vi "ParamControl.vi"(3 "Time Duration(ms)":i32, 4 "Packet":T1, 6 "Channel Array In":T2(array[cluster])) -> (1 "Ratio":dbl[](array[numeric]), 2 "Channel Array Out":T2(array[cluster]))   [LabVIEW 2014]
panel:
  out "Tmp Ratio":dbl[](array[numeric])
  out "Tmp Delay":dbl[](array[numeric])
  out "delta":dbl
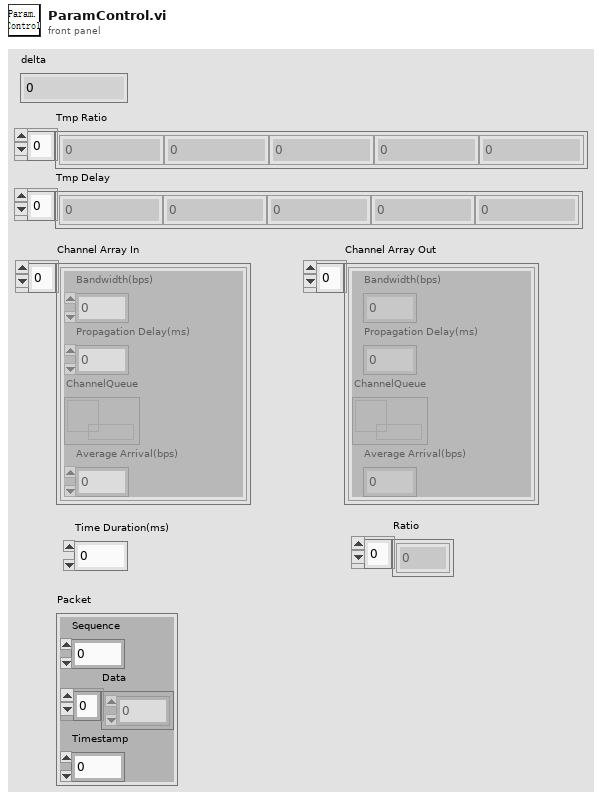
[diagram p1: front panel]
types:
  T1 = cluster{"Sequence":i32, "Data":u8[], "Timestamp":i32}
  T2 = cluster{"Bandwidth(bps)":i32, "Propagation Delay(ms)":i32, "ChannelQueue":refnum<queue>, "Average Arrival(bps)":dbl}[]
  T3 = cluster{"Bandwidth(bps)":i32, "Propagation Delay(ms)":i32, "ChannelQueue":refnum<queue>, "Average Arrival(bps)":dbl}
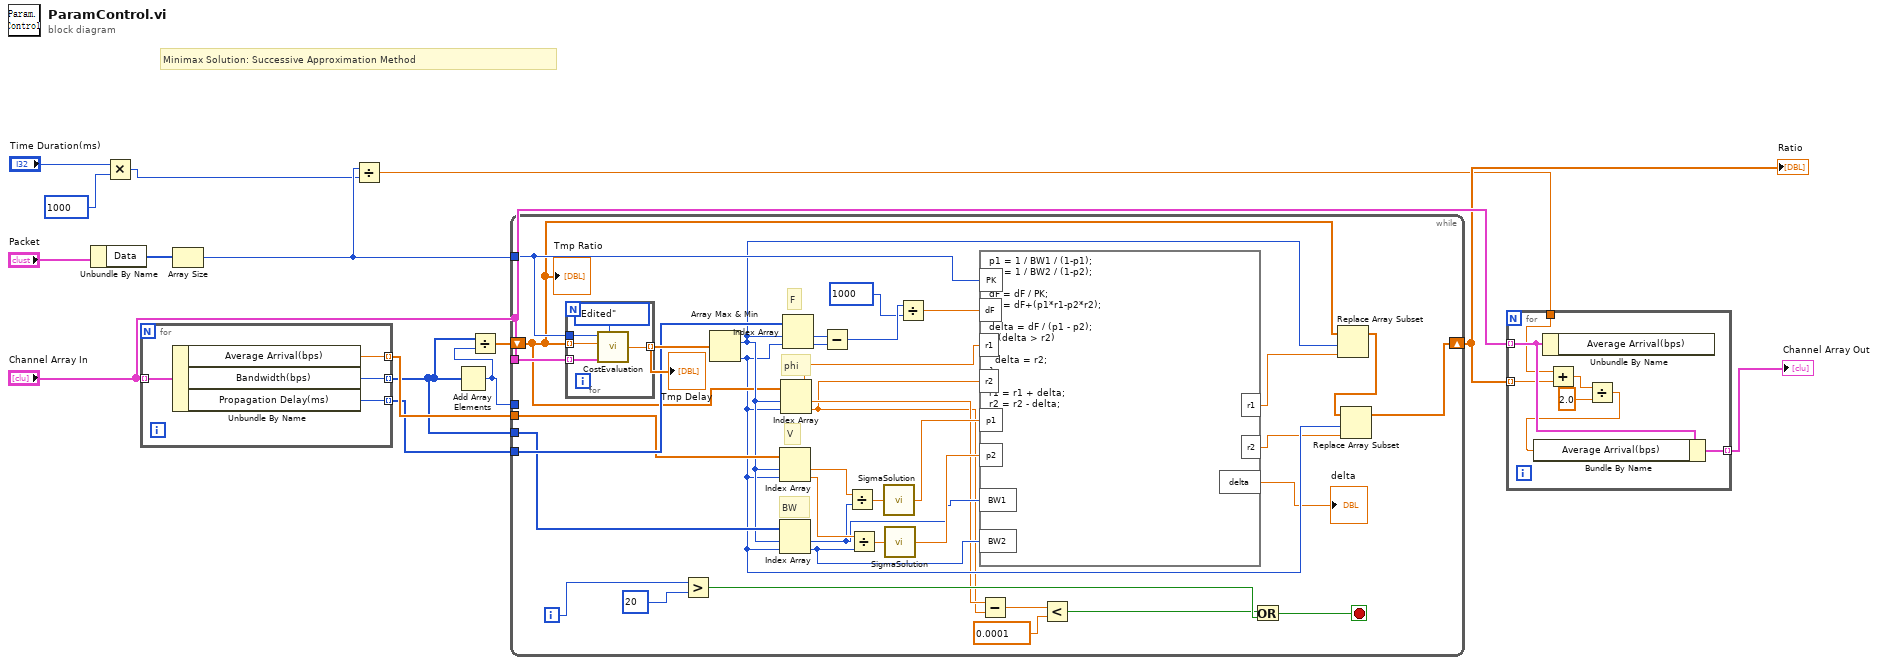
[diagram p0: block diagram]
diagram:
  # "Minimax Solution: Successive Approximation Method"
  n1 = Unbundle By Name("Packet") -> ("Data"=w15:u8[])
  n2 = Multiply(x="Time Duration(ms)", y=1000) -> (x*y=w5:i32)
  n3 = for {
    tunnel: "Channel Array In" -> [w19] mode=indexing
    tunnel: [w18] -> w13 mode=indexing
    tunnel: [w17] -> w12 mode=indexing
    tunnel: [w16] -> w11 mode=indexing
    n4 = Unbundle By Name(w19) -> ("Average Arrival(bps)"=w18:dbl, "Bandwidth(bps)"=w17:i32, "Propagation Delay(ms)"=w16:i32)
  }
  n5 = Array Size(array=w15) -> (size(s)=w6:i32)
  n6 = Divide(x=w6, y=w5) -> (x/y=w2:dbl)
  n7 = Add Array Elements(numeric array=w12) -> (sum=w10:i32)
  n8 = Divide(x=w12, y=w10) -> (x/y=w14:dbl[])
  n9 = while {
    tunnel: w6 -> [w40]
    tunnel: "Channel Array In" -> [w52]
    tunnel: w13 -> [w46]
    tunnel: w12 -> [w45]
    tunnel: w11 -> [w49]
    shift-right: [w28] -> w3
    shift-left: w14 -> [w33]
    tunnel: w10 -> [_]
    i -> [w55]
    stop <- w50 stop-if-true
    # "BW"
    # "V"
    # "phi"
    # "F"
    n10 = for {
      tunnel: w33 -> [w60] mode=indexing
      tunnel: w40 -> [w59]
      tunnel: w52 -> [w58] mode=indexing
      tunnel: [w57] -> w51 mode=indexing
      n11 = call "CostEvaluation.vi"("Packet Size"=w59, "Ratio"=w60, "Channel"=w58, "method"=enum16{"Edited", "original"}."Edited") -> ("delay(s)"=w57:dbl)  [unwired: 1 in]
    }
    "Tmp Delay" <- w51
    n12 = Greater?(x=w55, y=20) -> (0:w53:bool)
    n13 = Array Max & Min(array=w51) -> (max index (indices)=w34:i32, min index (indices)=w32:i32)  [unwired: 2 out]
    n14 = Index Array(array=w46, index #1=w34, index #2=w32) -> (element #1=w42:dbl, element #2=w41:dbl)
    n15 = Index Array(array=w45, index #1=w34, index #2=w32) -> (element #1=w36:i32, element #2=w35:i32)
    n16 = Index Array(array=w33, index #1=w34, index #2=w32) -> (element #1=w27:dbl, element #2=w26:dbl)
    n17 = Index Array(array=w49, index #1=w34, index #2=w32) -> (element #1=w47:i32, element #2=w48:i32)
    n18 = Subtract(x=w47, y=w48) -> (x-y=w22:i32)
    n19 = Divide(x=w42, y=w36) -> (x/y=w44:dbl)
    n20 = Divide(x=w41, y=w35) -> (x/y=w43:dbl)
    n21 = call "SigmaSolution.vi"("rou"=w44) -> ("sigma"=w39:dbl)
    n22 = call "SigmaSolution.vi"("rou"=w43) -> ("sigma"=w38:dbl)
    n23 = Divide(x=w22, y=1000) -> (x/y=w37:dbl)
    n24 = formula code="p1 = 1 / BW1 / (1-p1);\np2 = 1 / BW2 / (1-p2);\n\ndF = dF / PK;\ndF = dF+(p1*r1-p2*r2);\n\ndelta = dF / (p1 - p2);\nif (delta > r2)\n{\n  delta = r2;\n}\n\nr1 = r1 + delta;\nr2 = r2 - delta;"("PK"=w40, "dF"=w37, "p1"=w39, "p2"=w38, "BW1"=w36, "BW2"=w35, "r1"=w27, "r2"=w26) -> ("r1"=w31:dbl, "r2"=w29:dbl, "delta"=→"delta":dbl)
    n25 = Subtract(x=w27, y=w26) -> (x-y=w25:dbl)
    n26 = Less?(x=w25, y=0.0001) -> (x < y?=w23:bool)
    n27 = Or(x=w23, y=w53) -> (x .or. y?=w50:bool)
    n28 = Replace Array Subset(array=w33, new element=w31, index=w34) -> (w30:dbl[])
    n29 = Replace Array Subset(array=w30, new element=w29, index=w32) -> (w28:dbl[])
    "Tmp Ratio" <- w33
  }
  "Ratio" <- w3
  n30 = for {
    tunnel: "Channel Array In" -> [w67] mode=indexing
    tunnel: w3 -> [w64] mode=indexing
    tunnel: w2 -> [w65]
    tunnel: [w66] -> w1 mode=indexing
    n31 = Unbundle By Name(w67) -> ()  [unwired: 1 out]
    n32 = Add(x=w65, y=w64) -> (x+y=w63:dbl)
    n33 = Divide(x=w63, y=2.0) -> (x/y=w61:dbl)
    n34 = Bundle By Name(cluster=w67, "Average Arrival(bps)"=w61) -> (w66:T3)
  }
  "Channel Array Out" <- w1
